vi "CalculateColumnWidthsPx.vi"(6 "MinWidthAuto":i32=100, 9 "Column Sizes[]":i32[](array[numeric]), 10 "NumberOfColumns":i32=1, 11 "ContentWidth":i32) -> (3 "ColumnWidths (px)":i32[](array[numeric]))   [LabVIEW 2020, in "AdjMCLB.lvclass"]
uses:
  AdjMCLB.lvclass
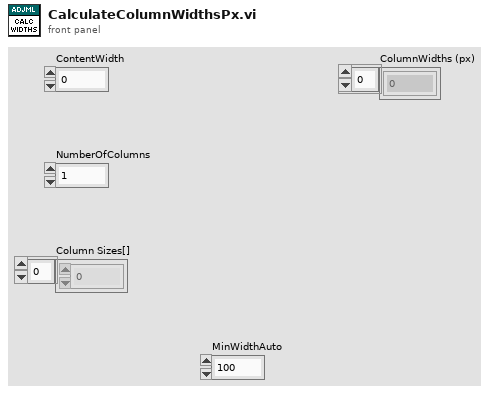
[diagram p1: front panel]
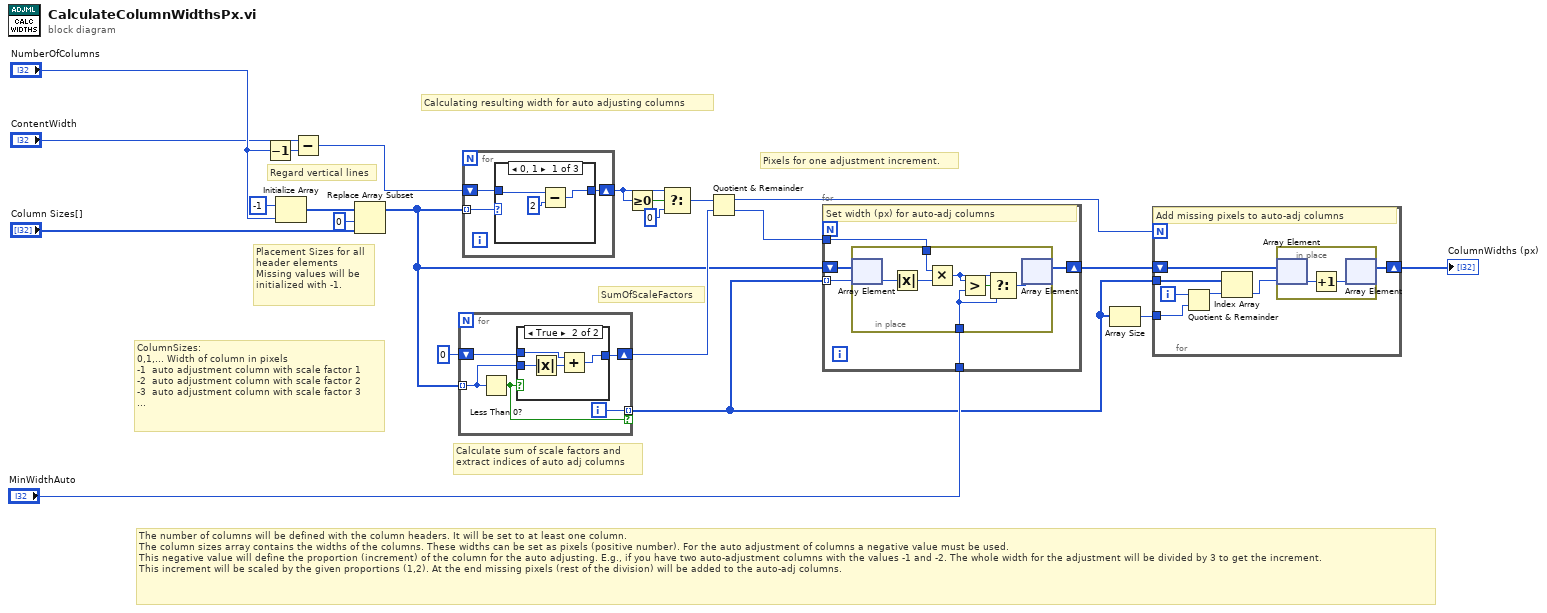
[diagram p0: block diagram]
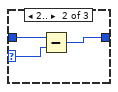
[diagram p3: hidden frame]
diagram:
  # "Pixels for one adjustment increment."
  # "The number of columns will be defined with the column headers. It will be set to at least one column.\nThe column sizes array contains the widths of the columns. These widths can be set as pixels (positive number). For the auto adjustment of columns a negative value must be used.\nThis negative value will define the proportion (increment) of the column for the auto adjusting. E.g., if you have two auto-adjustment columns with the values -1 and -2. The whole width for the adjustment will be divided by 3 to get the increment.\nThis increment will be scaled by the given proportions (1,2). At the end missing pixels (rest of the division) will be added to the auto-adj columns."
  # "Calculate sum of scale factors and\nextract indices of auto adj columns"
  # "Calculating resulting width for auto adjusting columns"
  # "SumOfScaleFactors"
  # "ColumnSizes:\n0,1,... Width of column in pixels\n-1  auto adjustment column with scale factor 1\n-2  auto adjustment column with scale factor 2\n-3  auto adjustment column with scale factor 3\n..."
  # "Placement Sizes for all\nheader elements\nMissing values will be\ninitialized with -1."
  # "Regard vertical lines"
  n1 = Decrement(x="NumberOfColumns") -> (x-1=w4:i32)
  n2 = Initialize Array(-1 ("element"), "NumberOfColumns") -> (w6:i32[])
  n3 = Subtract(x="ContentWidth", y=w4) -> (x-y=w9:i32)
  n4 = Replace Array Subset(array=w6, new element="Column Sizes[]", index=0) -> (w14:i32[])
  n5 = for {
    tunnel: w14 -> [w25] mode=indexing
    tunnel: [w27] -> w2 mode=indexing if=w26
    shift-right: [w23] -> w21
    shift-left: 0 -> [w24]
    i -> [w27]
    n6 = Less Than 0?(x=w25) -> (x < 0?=w26:bool)
    n7 = case shown="True" w26 {
      tunnel: w25 -> [_ w31]
      tunnel: w24 -> [w28 w30]
      tunnel: [w28 w29] -> w23
      frame False {
      }
      frame True {
        n8 = Absolute Value(x=w31) -> (abs(x)=w32:i32)
        n9 = Add(x=w30, y=w32) -> (x+y=w29:i32)
      }
    }
  }
  n10 = for {
    tunnel: w14 -> [w35] mode=indexing
    shift-right: [w33] -> w11
    shift-left: w9 -> [w34]
    n11 = case shown="0, 1" w35 {
      selector: w35 -> [_ w40 _]
      tunnel: w34 -> [w37 w41 w42]
      tunnel: [w38 w39 w42] -> w33
      frame 0, 1 {
        n12 = Subtract(x=w37, y=2) -> (x-y=w38:i32)
      }
      frame 2.. {
        n13 = Subtract(x=w41, y=w40) -> (x-y=w39:i32)
      }
      frame Default {
      }
    }
  }
  n14 = Greater Or Equal To 0?(x=w11) -> (x >= 0?=w10:bool)
  n15 = Select(t=w11, s=w10, f=0) -> (s? t:f=w13:i32)
  n16 = Quotient & Remainder(x=w13, y=w21) -> (x-y*floor(x/y)=w17:i32, floor(x/y)=w15:i32)
  n17 = for {
    shift-right: [w46] -> w16
    shift-left: w14 -> [w47]
    tunnel: w2 -> [w45] mode=indexing
    tunnel: w15 -> [w44]
    tunnel: "MinWidthAuto" -> [w43]
    # "Set width (px) for auto-adj columns"
    n18 = in-place {
      in-place-border: w44 -> [w52]
      in-place-border: w43 -> [w48]
      n19 = in-place-array #1(w47, w45) -> (w54:i32)
      n20 = Absolute Value(x=w54) -> (abs(x)=w53:i32)
      n21 = Multiply(x=w52, y=w53) -> (x*y=w50:i32)
      n22 = Greater?(x=w50, y=w48) -> (0:w51:bool)
      n23 = Select(t=w50, s=w51, f=w48) -> (s? t:f=w49:i32)
      n24 = in-place-array #1(w49) -> (w46:i32[])  [unwired: 1 out]
    }
  }
  n25 = Array Size(array=w2) -> (size(s)=w1:i32)
  n26 = for {
    N: w17 -> [_]
    shift-right: [w60] -> w18
    shift-left: w16 -> [w61]
    tunnel: w2 -> [w59]
    tunnel: w1 -> [w55]
    i -> [w57]
    # "Add missing pixels to auto-adj columns"
    n27 = Quotient & Remainder(x=w57, y=w55) -> (x-y*floor(x/y)=w56:i32)  [unwired: 1 out]
    n28 = Index Array(array=w59, index=w56) -> (element=w58:i32)
    n29 = in-place {
      n30 = in-place-array #2(w61, w58) -> (w63:i32)
      n31 = Increment(x=w63) -> (x+1=w62:i32)
      n32 = in-place-array #2(w62) -> (w60:i32[])  [unwired: 1 out]
    }
  }
  "ColumnWidths (px)" <- w18
